vi "Launcher.vi"   [LabVIEW 2015]
uses:
  Libraries/Audio Input/Audio Input.lvlib
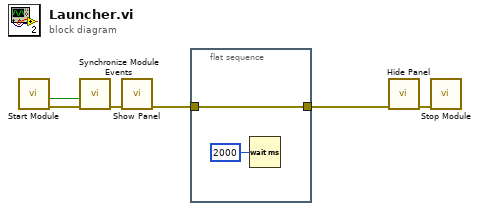
[diagram p0: block diagram]
diagram:
  n1 = call "Start Module.vi"() -> ("error out"=w6:errorcluster, "Wait for Event Sync?"=w3:bool)  [unwired: 8 in, 2 out]
  n2 = call "Synchronize Module Events.vi"("error in (no error)"=w6, "Wait for Event Sync?"=w3) -> ("error out"=w5:errorcluster)  [unwired: 9 in]
  n3 = call "Show Panel.vi"("error in (no error)"=w5) -> ("error out"=w1:errorcluster)  [unwired: 10 in]
  n4 = flat-sequence {
    tunnel: [w7] -> w2
    tunnel: w1 -> [w7]
    frame #0 {
      n5 = Wait (ms)(milliseconds to wait=u32 2000) -> ()  [unwired: 1 out]
    }
  }
  n6 = call "Hide Panel.vi"("error in (no error)"=w2) -> ("error out"=w4:errorcluster)  [unwired: 10 in]
  n7 = call "Stop Module.vi"("error in (no error)"=w4) -> ()  [unwired: 10 in, 1 out]
